vi "set_center.vi"(8 "error in (no error)":errorcluster, 10 "new center":refnum<class "SpaceVector.lvclass">, 11 "Box in":refnum<class "Box.lvclass">) -> (0 "error out":errorcluster, 3 "Box out":refnum<class "Box.lvclass">)   [LabVIEW 2010, in "Box.lvclass"]
uses:
  Box.lvclass
  SpaceVector/SpaceVector/SpaceVector.lvclass
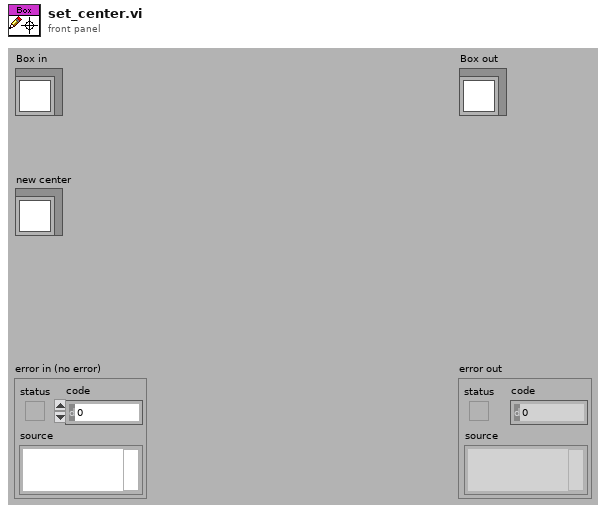
[diagram p1: front panel]
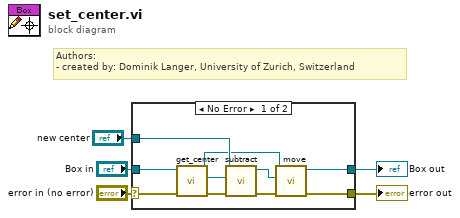
[diagram p0: block diagram]
diagram:
  # "Authors: \n- created by: Dominik Langer, University of Zurich, Switzerland"
  n1 = case shown="No Error" "error in (no error)" {
    selector: "error in (no error)" -> [w14 w17]
    tunnel: [w8 w17] -> w4
    tunnel: [w6 w16] -> w2
    tunnel: "Box in" -> [w15 w16]
    tunnel: "new center" -> [w13 _]
    frame No Error {
      n2 = call "get_center.vi"("error in (no error)"=w14, "Box in"=w15) -> ("error out"=w11:errorcluster, "center"=w12:refnum<class "SpaceVector.lvclass">, "Box out"=w7:refnum<class "Box.lvclass">)  [unwired: 7 in]
      n3 = call "subtract.vi"("error in (no error)"=w11, "subtrahend"=w12, "SpaceVector in"=w13) -> ("error out"=w9:errorcluster, "SpaceVector out"=w10:refnum<class "SpaceVector.lvclass">)  [unwired: 7 in]
      n4 = call "move.vi"("error in (no error)"=w9, "translation vector"=w10, "Box in"=w7) -> ("error out"=w8:errorcluster, "Box out"=w6:refnum<class "Box.lvclass">)  [unwired: 7 in]
    }
    frame Error {
    }
  }
  "error out" <- w4
  "Box out" <- w2
